vi "Acub.Start.vi"(5 "Autoshutdown? (T)":bool=TRUE, 8 "error in (no error)":errorcluster, 11 "NewTemplate in":refnum<class "Acub.lvclass">) -> (0 "error out":errorcluster, 1 "StartupHandshake out":refnum<class "RQMHStartup.lvclass">, 2 "_TemplateModule":cluster{"Broadcasts":T1, "Broadcasts":T2}, 3 "NewTemplate out":refnum<class "Acub.lvclass">)   [LabVIEW 2024, in "Acub.lvclass"]
uses:
  Acub.lvclass/Acub.ctl
  Acub.lvclass
  JQMHCore/Module/RQMHModule.lvclass
  Stopped.ctl
  Broadcast Events--cluster.ctl
  JQMHCore/Shared/Died.ctl
  JQMHCore/Shared/JQMHShared.lvlib
  JQMHCore/Module/StandardBroadcasts.ctl
  JQMHCore/Module/Started.ctl
  JQMHCore/JQMHStartup/RQMHStartup.lvclass
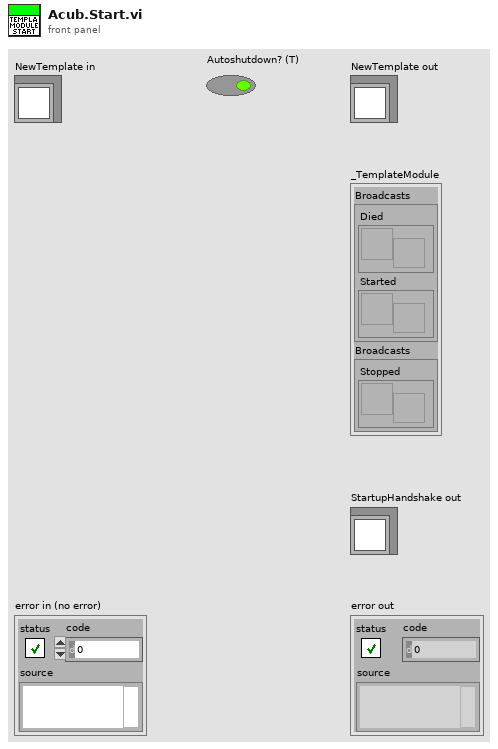
[diagram p1: front panel]
types:
  T1 = typedef "RQMHModule.lvclass/StandardBroadcasts.ctl" = cluster{"Died":refnum<user-event>, "Started":refnum<user-event>}
  T2 = typedef "Acub.lvclass/Broadcast Events--cluster.ctl" = cluster{"Stopped":refnum<user-event>}
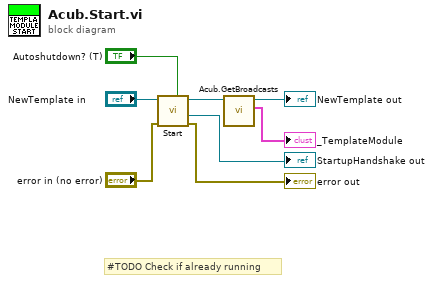
[diagram p0: block diagram]
diagram:
  # "#TODO Check if already running"
  n1 = call "Start.vi"("Autoshutdown? (T)"="Autoshutdown? (T)", "error in (no error)"="error in (no error)", "JQMHCore in"="NewTemplate in") -> ("error out"=→"error out":errorcluster, "StartupHandshake out"=→"StartupHandshake out":refnum<class "RQMHStartup.lvclass">, "JQMHCore out"=w4:refnum<class "Acub.lvclass">)  [unwired: 6 in]
  n2 = call "Acub.GetBroadcasts.vi"("NewTemplate in"=w4) -> ("TemplateModule"=→"_TemplateModule":cluster{"Broadcasts":T1, "Broadcasts":T2}, "NewTemplate out"=→"NewTemplate out":refnum<class "Acub.lvclass">)  [unwired: 9 in]
